vi "Dificult.vi"(8 "error in (no error)":errorcluster, 11 "Board_Game in":refnum<class "Board_Game.lvclass">) -> (0 "error out":errorcluster, 2 "Difficult":i32, 3 "Board_Game out":refnum<class "Board_Game.lvclass">)   [LabVIEW 2021, in "Board_Game.lvclass"]
uses:
  Board_Game.lvclass
  Board_Game.lvclass/Board_Game.ctl
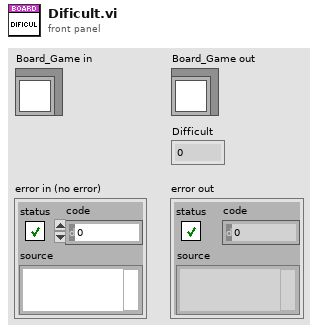
[diagram p1: front panel]
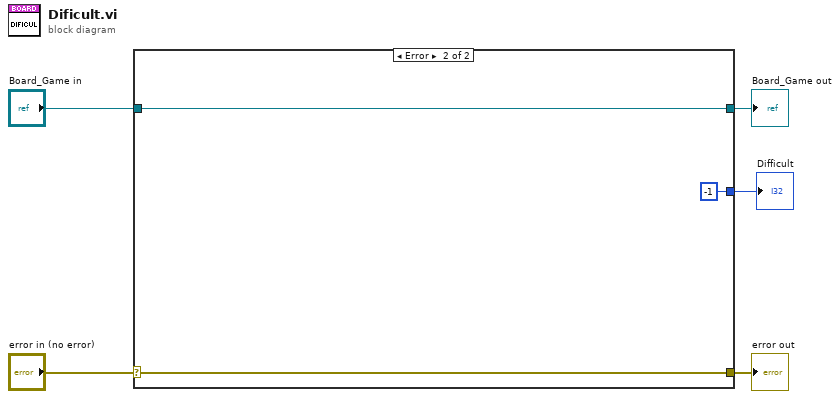
[diagram p0: block diagram]
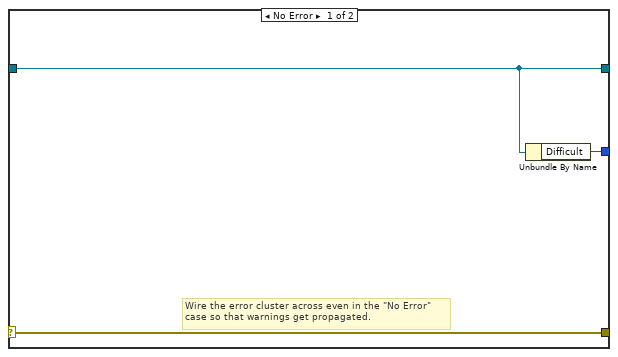
[diagram p2: hidden frame]
diagram:
  n1 = case shown="Error" "error in (no error)" {
    selector: "error in (no error)" -> [w8 w11]
    tunnel: [w8 w11] -> w4
    tunnel: [w7 w10] -> w2
    tunnel: "Board_Game in" -> [w7 w10]
    tunnel: [w6 -1 ("Difficult")] -> w1
    frame No Error {
      # "Wire the error cluster across even in the \"No Error\"\ncase so that warnings get propagated."
      n2 = Unbundle By Name(w7) -> ("Difficult"=w6:i32)
    }
    frame Error {
    }
  }
  "error out" <- w4
  "Board_Game out" <- w2
  "Difficult" <- w1
